vi "Compile Pattern.vi"(0 "Digital Pattern":string, 5 "Destination":path, 11 "error in (no error)":errorcluster, 12 "Delete Source File":bool=TRUE) -> (4 "Compiled Pattern Path":path, 15 "error out":errorcluster)   [LabVIEW 2018, in "MIPI RFFE API.lvlib"]
uses:
  MIPI RFFE API.lvlib
  <vilib>/regexp/Match Regular Expression.xnode
panel:
  out "standard output":string
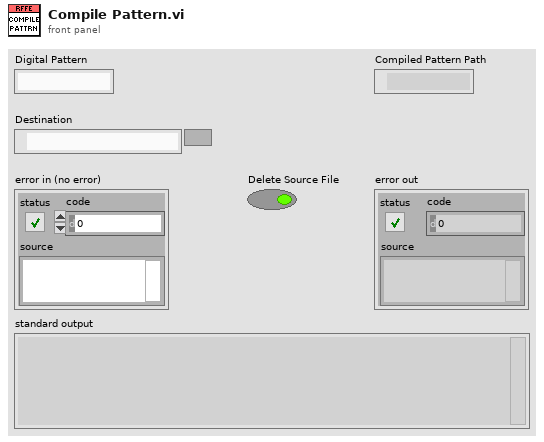
[diagram p1: front panel]
types:
  T1 = enum16{"open", "replace", "create", "open or create", "replace or create", "replace or create with confirmation"}
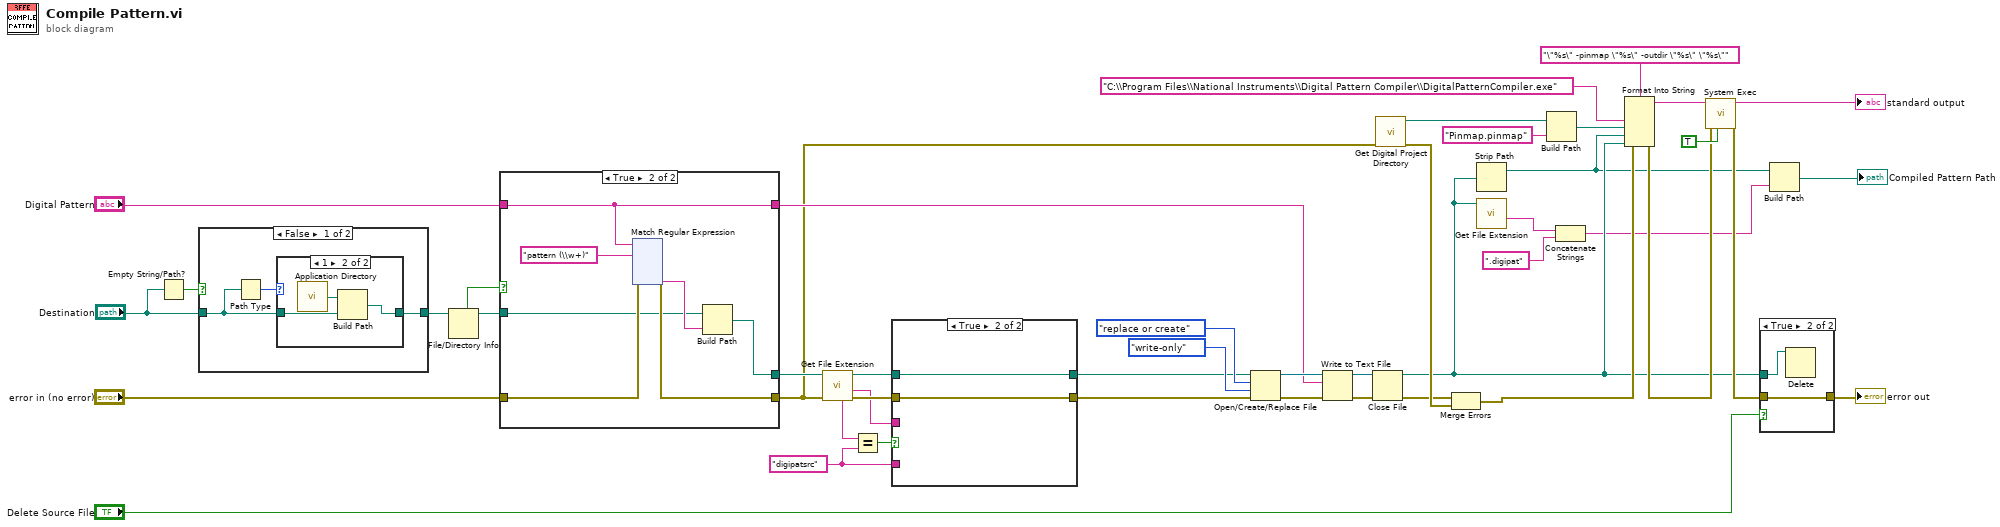
[diagram p0: block diagram]
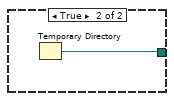
[diagram p3: hidden frame]
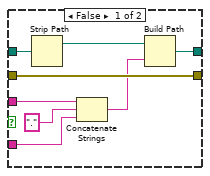
[diagram p5: hidden frame]
diagram:
  w2 = "digipatsrc" ("y")
  n1 = Empty String/Path?(string/path="Destination") -> (empty?=w16:bool)
  n2 = case shown="False" w16 {
    tunnel: "Destination" -> [w47 _]
    tunnel: [w46 w53] -> w15
    frame False {
      n3 = Path Type(1:w47) -> (0:w48:i16)
      n4 = case shown="1" w48 {
        tunnel: w47 -> [w49 w52]
        tunnel: [w49 w50] -> w46
        frame Default {
        }
        frame 1 {
          n5 = call <vilib>:"Application Directory.vi"() -> ("Application Directory"=w51:path)
          n6 = Build Path(base path=w51, name or relative path=w52) -> (appended path=w50:path)
        }
      }
    }
    frame True {
      n7 = Temporary Directory() -> (w53:path)
    }
  }
  n8 = File/Directory Info(path=w15) -> (path out=w14:path, directory=w13:bool)  [unwired: 1 in, 5 out]
  n9 = case shown="True" w13 {
    tunnel: [w54 w61] -> w9
    tunnel: "Digital Pattern" -> [w56 w57]
    tunnel: [w55 w60] -> w10
    tunnel: "error in (no error)" -> [w54 w59]
    tunnel: w14 -> [w55 w58]
    tunnel: [w56 w57] -> w24
    frame False {
    }
    frame True {
      n10 = xnode "Match Regular Expression"("input string"=w57, "regular expression"="pattern (\\w+)", "error in"=w59) -> ("error out"=w61:errorcluster, "submatch 1"=w63:string)  [unwired: 3 in, 4 out]
      n11 = Build Path(base path=w58, name or relative path=w63) -> (appended path=w60:path)
    }
  }
  n12 = call <vilib>:"Get File Extension.vi"("error in (no error)"=w9, "file"=w10) -> ("error out"=w6:errorcluster, "filename without extension"=w3:string, "dup file"=w4:path, "unmodified file extension"=w8:string)  [unwired: 5 in, 1 out]
  n13 = Equal?(x=w8, y=w2) -> (x = y?=w7:bool)
  n14 = case shown="True" w7 {
    tunnel: w6 -> [w187 w188]
    tunnel: [w187 w188] -> w5
    tunnel: w4 -> [w186 w189]
    tunnel: w3 -> [w185 _]
    tunnel: w2 -> [w183 _]
    tunnel: [w180 w189] -> w1
    frame False {
      n15 = Strip Path(path=w186) -> (stripped path=w182:path)  [unwired: 1 out]
      n16 = Concatenate Strings(w185, "." ("string"), w183) -> (w181:string)
      n17 = Build Path(base path=w182, name or relative path=w181) -> (appended path=w180:path)
    }
    frame True {
    }
  }
  n18 = Open/Create/Replace File(file path (use dialog)=w1, error in=w5, operation (0:open)=T1."replace or create", access (0:read/write)=enum16{"read/write", "read-only", "write-only"}."write-only") -> (refnum out=w29:refnum<file>, error out=w31:errorcluster)  [unwired: 2 in, 1 out]
  n19 = Write to Text File(file (use dialog)=w29, text=w24, error in=w31) -> (refnum out=w28:refnum<file>, error out=w30:errorcluster)  [unwired: 1 in, 1 out]
  n20 = Close File(refnum=w28, error in=w30) -> (path=w22:path, error out=w26:errorcluster)
  n21 = call "Get Digital Project Directory.vi"("error in (no error)"=w9) -> ("Digital Project Directory"=w34:path, "error out"=w27:errorcluster)  [unwired: 13 in]
  n22 = Merge Errors(w26, w27) -> (w23:errorcluster)
  n23 = Strip Path(path=w22) -> (stripped path=w21:path)  [unwired: 1 out]
  n24 = call <vilib>:"Get File Extension.vi"("file"=w22) -> ("filename without extension"=w20:string)  [unwired: 6 in, 4 out]
  n25 = Build Path(base path=w34, name or relative path="Pinmap.pinmap") -> (appended path=w33:path)
  n26 = Concatenate Strings(w20, ".digipat" ("string")) -> (w18:string)
  n27 = Format Into String(format string="\"%s\" -pinmap \"%s\" -outdir \"%s\" \"%s\"", error in=w23, "C:\\Program Files\\National Instruments\\Digital Pattern Compiler\\DigitalPatternCompiler.exe", w33, w21, w22) -> (resulting string=w37:string, error out=w36:errorcluster)  [unwired: 1 in]
  n28 = call <vilib>:"System Exec.vi"("run minimized? (F)"=TRUE, "error in (no error)"=w36, "command line"=w37) -> ("error out"=w32:errorcluster, "standard output"=→"standard output":string)  [unwired: 5 in, 2 out]
  n29 = case shown="True" "Delete Source File" {
    tunnel: w22 -> [_ w192]
    tunnel: w32 -> [w190 w191]
    tunnel: [w190 w191] -> w45
    frame False {
    }
    frame True {
      n30 = Delete(path (use dialog)=w192) -> ()  [unwired: 4 in, 3 out]
    }
  }
  "error out" <- w45
  n31 = Build Path(base path=w21, name or relative path=w18) -> (appended path=→"Compiled Pattern Path":path)
